vi "Get URI.vi"(6 "HTML Entity (F)":bool, 8 "error in (no error)":errorcluster, 11 "URI in":refnum<class "URI.lvclass">) -> (0 "error out":errorcluster, 2 "URI String":string, 3 "URI":refnum<class "URI.lvclass">)   [LabVIEW 2013, in "openURI.lvlib" / "URI.lvclass"]
uses:
  URI.lvclass
  URI.lvclass/URI.ctl
  Read scheme.vi
  Read host.vi
  Read port.vi
  Read username.vi
  Read password.vi
  Read fragment.vi
  utilities/isHEXDigit.vi
  components/path/Get path (absolute).vi
  <vilib>/Utility/error.llb/Trim Whitespace.vi
  openURI.lvlib
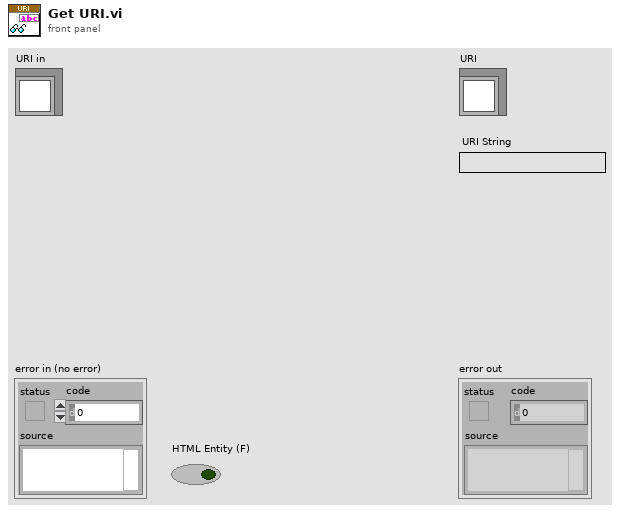
[diagram p1: front panel]
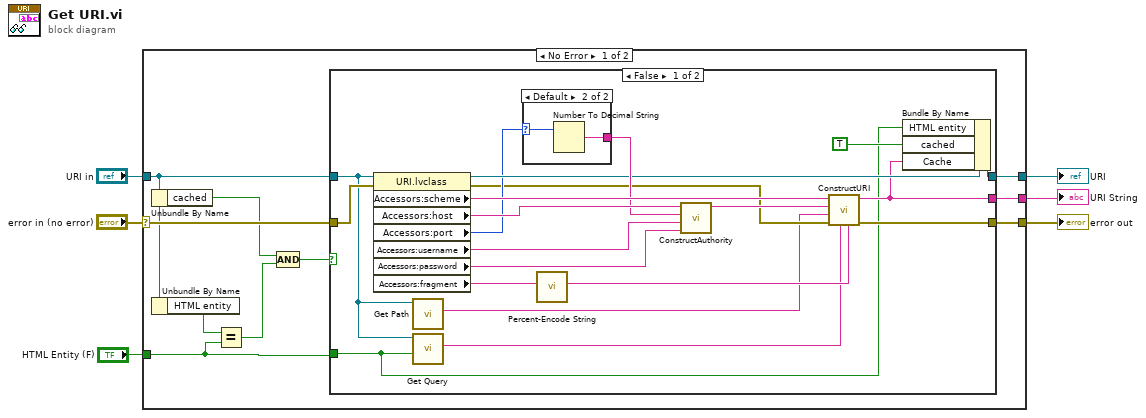
[diagram p0: block diagram]
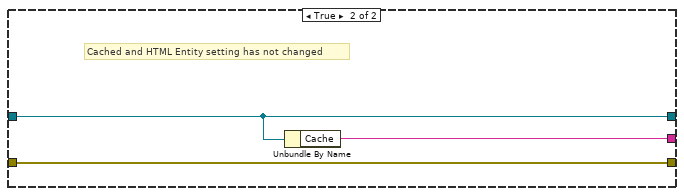
[diagram p3: hidden frame]
diagram:
  n1 = case shown="No Error" "error in (no error)" {
    selector: "error in (no error)" -> [w15 w43]
    tunnel: [w16 w43] -> w5
    tunnel: [w13 w42] -> w3
    tunnel: "URI in" -> [w10 w42]
    tunnel: [w14 _] -> w2
    tunnel: "HTML Entity (F)" -> [w8 _]
    frame No Error {
      n2 = Unbundle By Name(w10) -> ("cached"=w12:bool)
      n3 = Unbundle By Name(w10) -> ("HTML entity"=w9:bool)
      n4 = Equal?(x=w9, y=w8) -> (x = y?=w7:bool)
      n5 = Compound Arithmetic op=AND(w12, w7) -> (w11:bool)
      n6 = case shown="False" w11 {
        tunnel: [w30 w41] -> w16
        tunnel: w15 -> [w24 w41]
        tunnel: [w23 w39] -> w14
        tunnel: [w28 w40] -> w13
        tunnel: w10 -> [w19 w40]
        tunnel: w8 -> [w17 _]
        frame False {
          n7 = property class="URI.lvclass"(reference=w19, error in=w24) -> (reference out=w29:refnum<class "URI.lvclass">, error out=w25:errorcluster, "Accessors:scheme"=w36:string, "Accessors:host"=w34:string, "Accessors:port"=w26:u16, "Accessors:username"=w32:string, "Accessors:password"=w31:string, "Accessors:fragment"=w22:string)
          n8 = call "Get Path.vi"("URI in"=w19) -> ("path"=w20:string)  [unwired: 8 in, 2 out]
          n9 = call "Get Query.vi"("HTML Entity (F)"=w17, "URI in"=w19) -> ("query"=w18:string)  [unwired: 7 in, 2 out]
          n10 = case shown="Default" w26 {
            selector: w26 -> [_ w37]
            tunnel: [_ w38] -> w33
            frame 0 {
            }
            frame Default {
              n11 = Number To Decimal String(number=w37) -> (decimal integer string=w38:string)  [unwired: 1 in]
            }
          }
          n12 = call "Percent-Encode String.vi"("String"=w22) -> ("Pct-Encoded String"=w21:string)  [unwired: 10 in]
          n13 = call "ConstructAuthority.vi"("password"=w31, "username"=w32, "port"=w33, "host"=w34) -> ("authority"=w35:string)  [unwired: 7 in]
          n14 = call "ConstructURI.vi"("fragment"=w21, "query"=w18, "error in"=w25, "path component"=w20, "authority"=w35, "scheme"=w36) -> ("error out"=w30:errorcluster, "URI"=w23:string)  [unwired: 4 in]
          n15 = Bundle By Name(cluster=w29, "HTML entity"=w17, "cached"=TRUE, "Cache"=w23) -> (w28:refnum<class "URI.lvclass">)
        }
        frame True {
          # "Cached and HTML Entity setting has not changed"
          n16 = Unbundle By Name(w40) -> ("Cache"=w39:string)
        }
      }
    }
    frame Error {
    }
  }
  "error out" <- w5
  "URI" <- w3
  "URI String" <- w2
